vi "Send Task Status Update.vi"(8 "error in (no error)":errorcluster, 9 "Status":T1=enum."Added", 10 "Task Name":string, 11 "BuildWorker in":refnum<class "BuildWorker.lvclass">) -> (0 "error out":errorcluster, 3 "BuildWorker out":refnum<class "BuildWorker.lvclass">)   [LabVIEW 2017, in "BuildWorker.lvlib" / "BuildWorker.lvclass"]
uses:
  BuildWorker.lvclass
  WebSocket Server/Actors/WebSocket Client/WebSocket Client Messages/Send Message Msg/Send Message Msg.lvclass
  BuildWorker Messages/Update Task List Msg/Update Task List Msg.lvclass
  <vilib>/ActorFramework/Actor/Actor.lvclass
  Classes/Status/Status.lvclass
  Classes/Task Status/Task Status.lvclass
  Volumes/Data/Users/benji667/Git/BuildFarm/BuildWorker/Classes/Status/Status.lvclass
  Classes/Task/Task.lvclass
  Applications/National Instruments/LabVIEW 2017 64-bit/vi.lib/ActorFramework/Actor/Actor.lvclass
  Classes/Task/Status.ctl
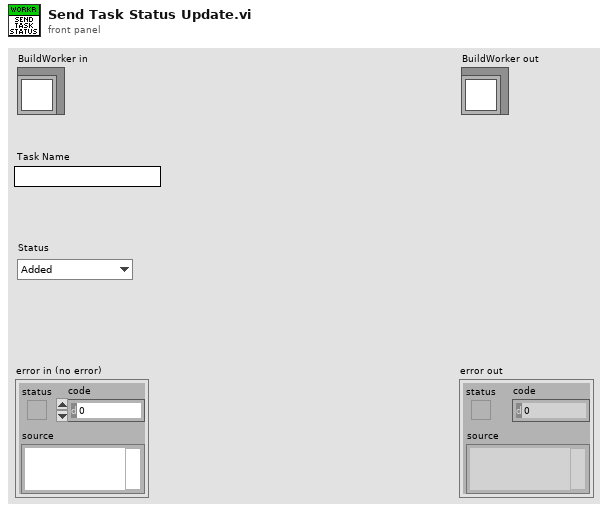
[diagram p1: front panel]
types:
  T1 = typedef "Task Interface.lvlib/Task.lvclass/Status.ctl" = enum16{"Created", "Added", "Pending", "Queued", "Processing", "Cleaning", "Building", "Finished", "Failed", "Removed", "Not found"}
  T2 = typedef "Task.lvclass/Status.ctl" = enum16{"Created", "Added", "Pending", "Queued", "Processing", "Cleaning", "Building", "Finished", "Failed", "Removed", "Not found"}
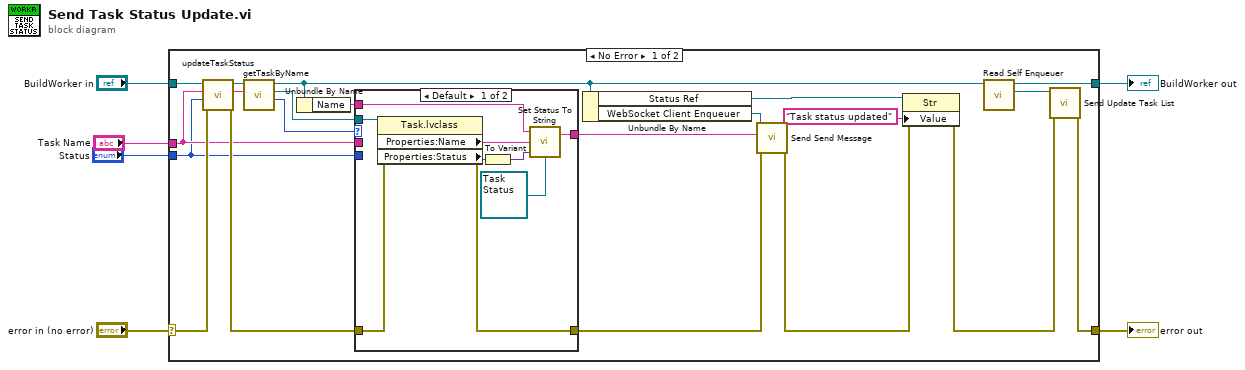
[diagram p0: block diagram]
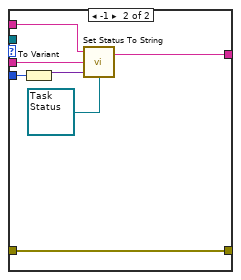
[diagram p2: hidden frame]
diagram:
  n1 = case shown="No Error" "error in (no error)" {
    selector: "error in (no error)" -> [w23 w43]
    tunnel: [w18 w43] -> w5
    tunnel: [w8 w42] -> w3
    tunnel: "BuildWorker in" -> [w24 w42]
    tunnel: "Task Name" -> [w15 _]
    tunnel: "Status" -> [w14 _]
    frame No Error {
      n2 = call "updateTaskStatus.vi"("error in (no error)"=w23, "Status"=w14, "Task Name"=w15, "BuildWorker in"=w24) -> ("error out"=w20:errorcluster, "BuildWorker out"=w22:refnum<class "BuildWorker.lvclass">)  [unwired: 6 in]
      n3 = call "getTaskByName.vi"("Task Name"=w15, "BuildWorker in"=w22) -> ("index of element"=w16:i32, "Task"=w21:refnum<class "Task.lvclass">, "BuildWorker out"=w8:refnum<class "BuildWorker.lvclass">)  [unwired: 7 in]
      n4 = Unbundle By Name(w8) -> ("Name"=w7:string)
      n5 = case shown="Default" w16 {
        tunnel: w21 -> [w34 _]
        tunnel: w20 -> [w30 w38]
        tunnel: [w29 w38] -> w10
        tunnel: w15 -> [_ w41]
        tunnel: w14 -> [_ w40]
        tunnel: [w31 w39] -> w11
        tunnel: w7 -> [w27 w36]
        frame Default {
          n6 = property class="Task.lvclass"(reference=w34, error in=w30) -> (error out=w29:errorcluster, "Properties:Name"=w33:string, "Properties:Status"=w32:T2)  [unwired: 1 out]
          n7 = To Variant(anything=w32) -> (Variant=w26:variant)
          n8 = call "Set Status To String.vi"("Status type"=refnum<class "Task Status.lvclass"> refnum ("Task Status.lvclass"), "Status"=w26, "Item Name"=w33, "Sender"=w27) -> ("data string"=w31:string)  [unwired: 1 in]
        }
        frame -1 {
          n9 = To Variant(anything=w40) -> (Variant=w35:variant)
          n10 = call "Set Status To String.vi"("Status type"=refnum<class "Task Status.lvclass"> refnum ("Task Status.lvclass"), "Status"=w35, "Item Name"=w41, "Sender"=w36) -> ("data string"=w39:string)  [unwired: 1 in]
        }
      }
      n11 = Unbundle By Name(w8) -> ("Status Ref"=w13:refnum<vi>, "WebSocket Client Enqueuer"=w12:refnum<class "Message Enqueuer.lvclass">)
      n12 = call "Send Send Message.vi"("error in (no error)"=w10, "Message"=w11, "Message Enqueuer in"=w12) -> ("error out"=w9:errorcluster)  [unwired: 7 in, 1 out]
      n13 = property class="Str"(reference=w13, error in=w9, "Value"="Task status updated") -> (error out=w17:errorcluster)  [unwired: 1 out]
      n14 = call <vilib>:"Read Self Enqueuer.vi"("Actor"=w8) -> ("Self Enqueuer"=w19:refnum<class "Message Enqueuer.lvclass">)  [unwired: 10 in]
      n15 = call "Send Update Task List.vi"("error in (no error)"=w17, "Message Enqueuer in"=w19) -> ("error out"=w18:errorcluster)  [unwired: 8 in, 1 out]
    }
    frame Error {
    }
  }
  "error out" <- w5
  "BuildWorker out" <- w3
